vi "fgv_Z planes.vi"(8 "error in (no error)":errorcluster, 9 "Motor Z planes":dbl[](array[numeric]), 10 "AOL Z Planes":dbl[](array[numeric]), 11 "Function":enum16{"Intialize", "Write", "Read", "Clear"}(ring)) -> (0 "error out":errorcluster, 1 "Motor Z planes":dbl[](array[numeric]), 2 "AOL Z Planes":dbl[](array[numeric]))   [LabVIEW 2020]
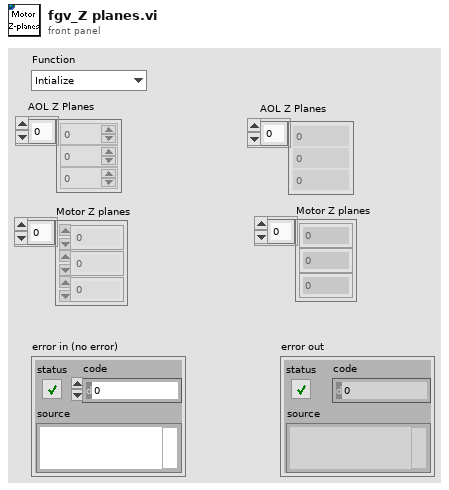
[diagram p1: front panel]
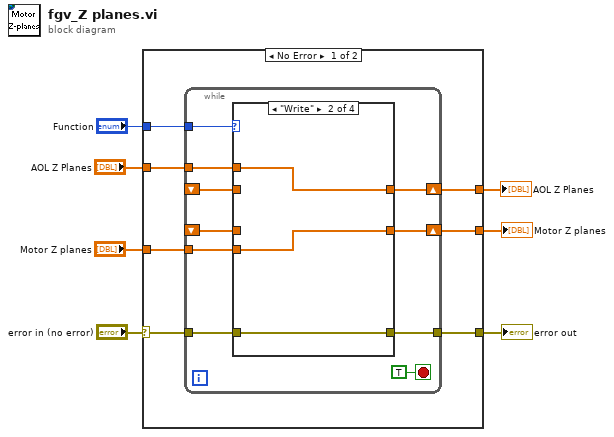
[diagram p0: block diagram]
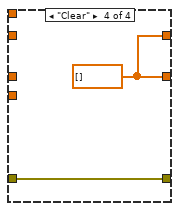
[diagram p4: hidden frame]
diagram:
  n1 = case shown="No Error" "error in (no error)" {
    selector: "error in (no error)" -> [w11 w38]
    tunnel: [w12 w38] -> w6
    tunnel: "Function" -> [w14 _]
    tunnel: "Motor Z planes" -> [w13 w37]
    tunnel: [w10 w37] -> w4
    tunnel: "AOL Z Planes" -> [w9 w36]
    tunnel: [w8 w36] -> w1
    frame No Error {
      n2 = while {
        tunnel: w14 -> [w23]
        tunnel: w13 -> [w22]
        shift-right: [w21] -> w10
        shift-left: _ -> [w20]
        tunnel: [w18] -> w12
        tunnel: w11 -> [w19]
        tunnel: w9 -> [w17]
        shift-right: [w16] -> w8
        shift-left: _ -> [w15]
        stop <- TRUE stop-if-true
        n3 = case shown="\"Write\"" w23 {
          tunnel: [w27 w30 w33 w34] -> w21
          tunnel: w22 -> [_ w30 _ _]
          tunnel: w20 -> [w27 _ w33 _]
          tunnel: [w26 w29 w32 w35] -> w18
          tunnel: w19 -> [w26 w29 w32 w35]
          tunnel: w17 -> [_ w28 _ _]
          tunnel: [w25 w28 w31 w34] -> w16
          tunnel: w15 -> [w25 _ w31 _]
          frame "Intialize", Default {
          }
          frame "Write" {
          }
          frame "Read" {
          }
          frame "Clear" {
            w34 = dbl[] [] ("Motor Z planes")
          }
        }
      }
    }
    frame Error {
    }
  }
  "error out" <- w6
  "Motor Z planes" <- w4
  "AOL Z Planes" <- w1
